vi "Vision Processing.vi"(4 "error in (no error)":errorcluster, 7 "Image Size":T3=enum."320x240") -> ()   [LabVIEW 2015]
uses:
  Vision Support Code/Camera Types.ctl
  <vilib>/Rock Robotics/WPI/Camera/WPI_CameraImageSize.ctl
  <vilib>/Rock Robotics/WPI/Camera/WPI_CameraExposure Values.ctl
  <vilib>/Rock Robotics/WPI/Camera/WPI_CameraFrameRate.ctl
  <vilib>/Rock Robotics/WPI/Camera/WPI_CameraWhite Balance Values.ctl
  <vilib>/Rock Robotics/Network Tables/NT Read Boolean.vi
  Robot Global Data.vi
  Global Variables/Vision Processing Data.vi
  <vilib>/vision/NI_Vision_Development_Module.lvlib
panel:
  out "Highest Avg Score":dbl
  in  "Min Score Threshold":i32=75
  out "Detected Targets":T1(array[cluster]) {"Normalized Rect"."Numeric 5" format="%#_2g"; "Normalized Rect"."Numeric 3" format="%#_2g"; "Normalized Rect"."Numeric 2" format="%#_2g"; "Normalized Rect"."Numeric" format="%#_2g"}
  out "Sorted Particle Scores":T2(array[cluster]) {"Moment Factor" format="%#_3g"; "Aspect Ratio" format="%#_3g"; "Area to CH" format="%#_3g"; "X" format="%#_3g"; "Y" format="%#_3g"}
  in  "Display Original":bool=TRUE
  in  "Display Mask":bool=TRUE
  out "fps":dbl
  in  "Emphasize Limit Tests":bool=TRUE
  in  "Camera Type":T4=enum."MS HD3000 square"
  in  "Aspect Fudge Factor":dbl=1.0
  in  "Score Threshold":dbl=75.0
  out "ms to process":u32
  out "Qualified Particles":i32
  in  "LED Color":T5={"Hue"={75.0, 175.0}, "Sat"={0.0, 255.0}, "Val"={50.0, 255.0}} {"Hue" scale=0.0..255.0 scale format="%#_3g"}
  out "Masked":T6(plugin-control)
  out "Original Image":T6(plugin-control)
  # "Density Profile"
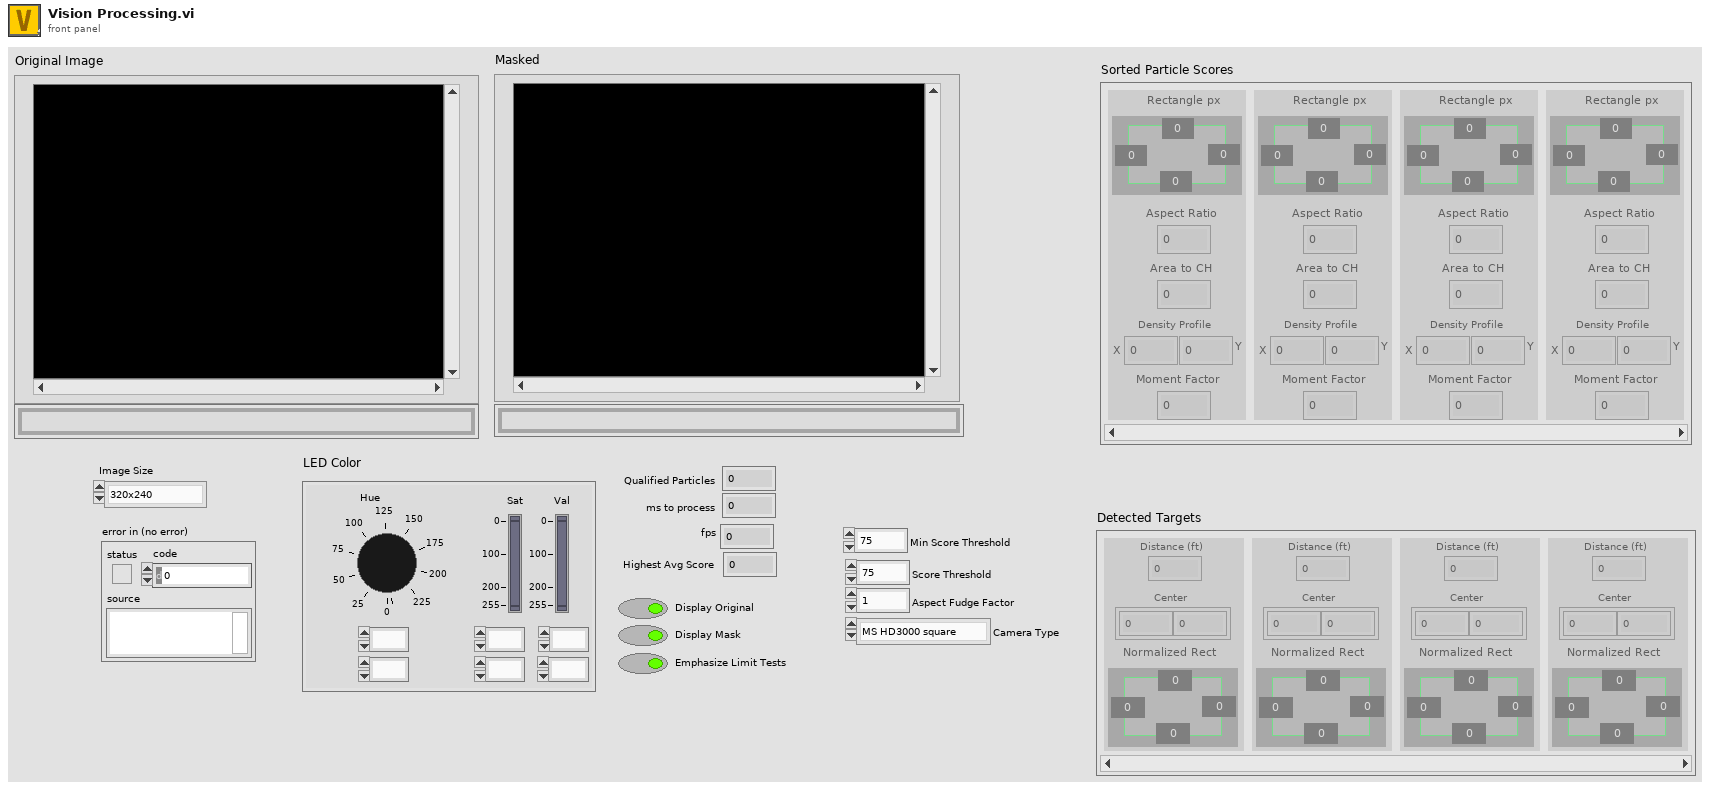
[diagram p1: front panel]
types:
  T1 = cluster{"Distance (ft)":dbl, "Center":cluster{dbl, dbl}, "Normalized Rect":cluster{"Numeric":dbl, "Numeric 2":dbl, "Numeric 3":dbl, "Numeric 5":dbl}}[]
  T2 = cluster{"Rectangle px":cluster{"Numeric":dbl, "Numeric 2":dbl, "Numeric 3":dbl, "Numeric 5":dbl}, "Aspect Ratio":dbl, "Area to CH":dbl, "X":dbl, "Y":dbl, "Moment Factor":dbl}[]
  T3 = typedef "WPI_CameraImageSize.ctl" = enum16{"640x480", "320x240", "160x120", "Custom"}
  T4 = typedef "Camera Types.ctl" = enum16{"206", "1011", "1013", "MS HD3000 square", "MS HD3000 640x480"}
  T5 = cluster{"Hue":cluster{dbl, dbl}, "Sat":cluster{dbl, dbl}, "Val":cluster{dbl, dbl}}
  T6 = typedef "IMAQ Image.ctl" = refnum<image>
  T7 = typedef "WPI_CameraWhite Balance Values.ctl" = enum16{"Auto", "Fixed indoor", "Fixed outdoor 1", "Fixed outdoor 2", "Fixed fluorescent 1", "Fixed fluorescent 2", "Hold current", "Custom"}
  T8 = typedef "WPI_CameraFrameRate.ctl" = u32
  T9 = typedef "WPI_CameraExposure Values.ctl" = enum16{"Auto", "Flicker-free 50 Hz", "Flicker-free 60 Hz", "Hold current", "Custom"}
  T10 = typedef "Particle Parameters" = i32
  T11 = typedef "Image Type" = u32
  T12 = typedef "WPI_CameraDevRef.ctl" = cluster{"Camera Address":string, "CameraStatus":errorcluster}
  T13 = cluster{"Bounding box":cluster{"left":dbl, "top":dbl, "right":dbl, "bottom":dbl}, "Aspect Ratio":dbl, "Area to CH":dbl, "X Mask":dbl, "Y Mask":dbl, "Moment":dbl}[]
  T14 = cluster{"Rectangle":cluster{"Numeric":dbl, "Numeric 2":dbl, "Numeric 3":dbl, "Numeric 5":dbl}, "L":dbl, "Area to CH":dbl, "X":dbl, "Y":dbl, "Moment Factor":dbl}[]
  T15 = cluster{"Distance (ft)":dbl, "Center":cluster{dbl, dbl}, "Normalized Rect":cluster{"Numeric":dbl, "Numeric 2":dbl, "Numeric 3":dbl, "Numeric 5":dbl}}
  T16 = cluster{"Rectangle":cluster{"Numeric":dbl, "Numeric 2":dbl, "Numeric 3":dbl, "Numeric 5":dbl}, "L":dbl, "Area to CH":dbl, "X":dbl, "Y":dbl, "Moment Factor":dbl}
  T17 = cluster{"Numeric":dbl, "Numeric 2":dbl, "Numeric 3":dbl, "Numeric 5":dbl}
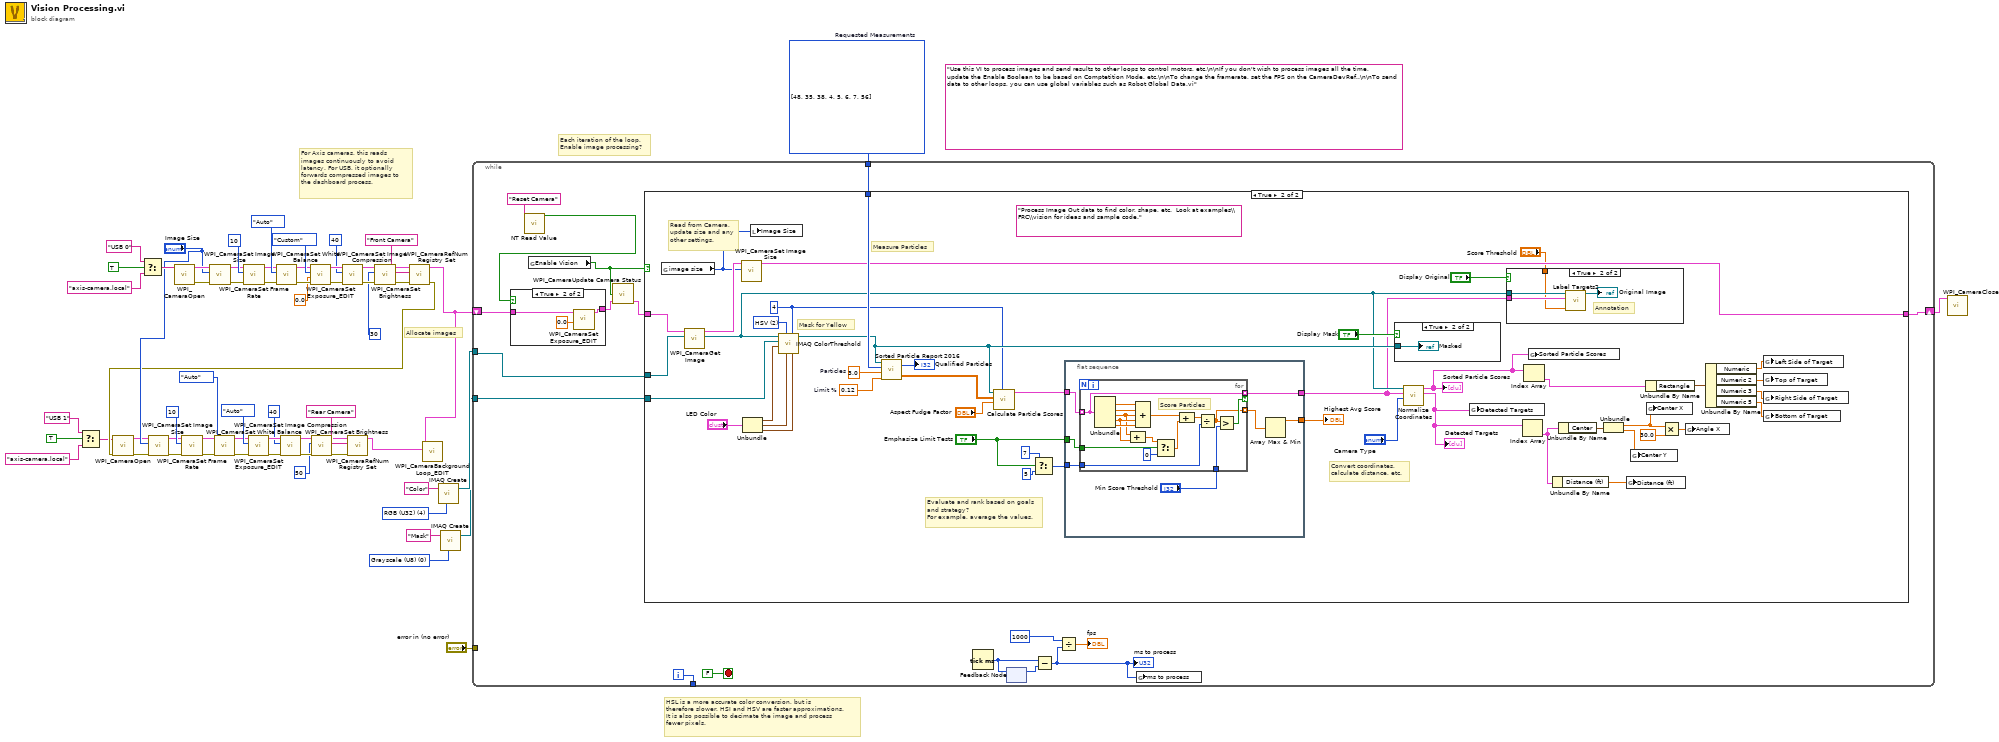
[diagram p0: block diagram]
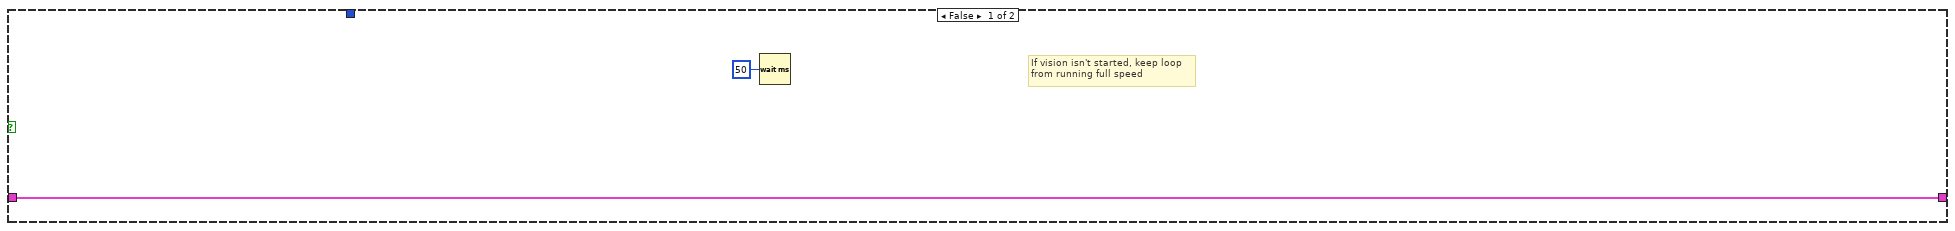
[diagram p3: hidden frame]
diagram:
  (unwired) "Use this VI to process images and send results to other loops to control motors, etc.\n\nIf you don't wish to process images all the time, update the Enable Boolean to be based on Comptetition Mode, etc.\n\nTo change the framerate, set the FPS on the CameraDevRef..\n\nTo send data to other loops, you can use global variables such as Robot Global Data.vi"
  w56 = T10[] [48, 35, 38, 4, 5, 6, 7, 56] items=["Center of Mass X", "Center of Mass Y", "First Pixel X", "First Pixel Y", "Bounding Rect Left", "Bounding Rect Top", "Bounding Rect Right", "Bounding Rect Bottom", "Max Feret Diameter Start X", "Max Feret Diameter Start Y", "Max Feret Diameter End X", "Max Feret Diameter End Y", "Max Horiz. Segment Length Left", "Max Horiz. Segment Length Right", "Max Horiz. Segment Length Row", "-", "Bounding Rect Width", "Bounding Rect Height", "Bounding Rect Diagonal", "Perimeter", "Convex Hull Perimeter", "Holes' Perimeter", "Max Feret Diameter", "Equivalent Ellipse Major Axis", "Equivalent Ellipse Minor Axis", "Equivalent Ellipse Minor Axis (Feret)", "Equivalent Rect Long Side", "Equivalent Rect Short Side", "Equivalent Rect Diagonal", "Equivalent Rect Short Side (Feret)", "Average Horiz. Segment Length", "Average Vert. Segment Length", "Hydraulic Radius", "Waddel Disk Diameter", "-", "Area", "Holes' Area", "Particle & Holes' Area", "Convex Hull Area", "Image Area", "-", "Number of Holes", "Number of Horiz. Segments", "Number of Vert. Segments", "-", "Orientation", "Max Feret Diameter Orientation", "-", "% Area/Image Area", "% Area/(Particle & Holes' Area)", "Ratio of Equivalent Ellipse Axes", "Ratio of Equivalent Rect Sides", "-", "Elongation Factor", "Compactness Factor", "Heywood Circularity Factor", "Type Factor", "-", "Sum X", "Sum Y", "Sum XX", "Sum XY", "Sum YY", "Sum XXX", "Sum XXY", "Sum XYY", "Sum YYY", "-", "Moment of Inertia XX", "Moment of Inertia XY", "Moment of Inertia YY", "Moment of Inertia XXX", "Moment of Inertia XXY", "Moment of Inertia XYY", "Moment of Inertia YYY", "Norm. Moment of Inertia XX", "Norm. Moment of Inertia XY", "Norm. Moment of Inertia YY", "Norm. Moment of Inertia XXX", "Norm. Moment of Inertia XXY", "Norm. Moment of Inertia XYY", "Norm. Moment of Inertia YYY", "Hu Moment 1", "Hu Moment 2", "Hu Moment 3", "Hu Moment 4", "Hu Moment 5", "Hu Moment 6", "Hu Moment 7"]  # Requested Measurements
  w59 = T11 0 items=["Grayscale (U8)", "Grayscale (I16)", "Grayscale (SGL)", "Complex (CSG)", "RGB (U32)", "HSL (U32)", "RGB (U64)", "Grayscale (U16)"] ("Image Type")
  w61 = T11 4 items=["Grayscale (U8)", "Grayscale (I16)", "Grayscale (SGL)", "Complex (CSG)", "RGB (U32)", "HSL (U32)", "RGB (U64)", "Grayscale (U16)"] ("Image Type")
  # "Each iteration of the loop,\nEnable image processing?"
  # "HSL is a more accurate color conversion, but is\ntherefore slower. HSI and HSV are faster approximations.\nIt is also possible to decimate the image and process\nfewer pixels."
  # "For Axis cameras, this reads\nimages continuously to avoid\nlatency. For USB, it optionally\nforwards compressed images to\nthe dashboard process."
  # "Allocate images"
  n1 = Select(t="USB 1" ("format string"), s=TRUE ("dot notation? (F)"), f="axis-camera.local" ("format string")) -> (s? t:f=w25:string)
  n2 = Select(t="USB 0" ("format string"), s=TRUE ("dot notation? (F)"), f="axis-camera.local" ("format string")) -> (s? t:f=w55:string)
  n3 = call <vilib>:"WPI_CameraOpen.vi"("Camera Address"=w55) -> ("error out"=w43:errorcluster, "CameraDevRef"=w42:T12)  [unwired: 1 in, 8 out]
  n4 = call <vilib>:"WPI_CameraSet Image Size.vi"("error in (no error)"=w43, "Image Size"="Image Size", "CameraDevRef"=w42) -> ("error out"=w44:errorcluster, "CameraDevRef Out"=w41:T12)  [unwired: 1 in, 6 out]
  n5 = call <vilib>:"WPI_CameraSet Frame Rate.vi"("error in (no error)"=w44, "Frame Rate (fps)"=T8 10, "CameraDevRef"=w41) -> ("error out"=w45:errorcluster, "CameraDevRef Out"=w39:T12)  [unwired: 7 out]
  n6 = call <vilib>:"WPI_CameraSet White Balance.vi"("error in (no error)"=w45, "White Balance"=WPI_CameraWhite_Balance_Values."Auto", "CameraDevRef"=w39) -> ("error out"=w46:errorcluster, "CameraDevRef Out"=w40:T12)  [unwired: 1 in, 6 out]
  n7 = call "WPI_CameraSet Exposure_EDIT.vi"("error in (no error)"=w46, "Exposure (%)"=0.0, "Exposure"=WPI_CameraExposure_Values."Custom", "CameraDevRef"=w40) -> ("error out"=w47:errorcluster, "CameraDevRef Out"=w37:T12)  [unwired: 6 out]
  n8 = call <vilib>:"WPI_CameraSet Image Compression.vi"("error in (no error)"=w47, "Compression"=40, "CameraDevRef"=w37) -> ("error out"=w48:errorcluster, "CameraDevRef Out"=w38:T12)  [unwired: 7 out]
  n9 = call <vilib>:"WPI_CameraSet Brightness.vi"("error in (no error)"=w48, "Brightness"=30, "CameraDevRef"=w38) -> ("error out"=w49:errorcluster, "CameraDevRef Out"=w31:T12)  [unwired: 7 out]
  n10 = call <vilib>:"WPI_CameraRefNum Registry Set.vi"("error in (no error)"=w49, "refnum name"="Front Camera", "CameraDevRef"=w31) -> ("error out"=w28:errorcluster, "CameraDevRef"=w26:T12)  [unwired: 1 in, 6 out]
  n11 = call <vilib>:"WPI_CameraOpen.vi"("error in (no error)"=w28, "Camera Address"=w25) -> ("error out"=w14:errorcluster, "CameraDevRef"=w13:T12)  [unwired: 8 out]
  n12 = call <vilib>:"WPI_CameraSet Image Size.vi"("error in (no error)"=w14, "Image Size"="Image Size", "CameraDevRef"=w13) -> ("error out"=w15:errorcluster, "CameraDevRef Out"=w12:T12)  [unwired: 1 in, 6 out]
  n13 = call <vilib>:"WPI_CameraSet Frame Rate.vi"("error in (no error)"=w15, "Frame Rate (fps)"=T8 10, "CameraDevRef"=w12) -> ("error out"=w16:errorcluster, "CameraDevRef Out"=w10:T12)  [unwired: 7 out]
  n14 = call <vilib>:"WPI_CameraSet White Balance.vi"("error in (no error)"=w16, "White Balance"=WPI_CameraWhite_Balance_Values."Auto", "CameraDevRef"=w10) -> ("error out"=w17:errorcluster, "CameraDevRef Out"=w11:T12)  [unwired: 1 in, 6 out]
  n15 = call "WPI_CameraSet Exposure_EDIT.vi"("error in (no error)"=w17, "Exposure"=WPI_CameraExposure_Values."Auto", "CameraDevRef"=w11) -> ("error out"=w18:errorcluster, "CameraDevRef Out"=w8:T12)  [unwired: 1 in, 6 out]
  n16 = call <vilib>:"WPI_CameraSet Image Compression.vi"("error in (no error)"=w18, "Compression"=40, "CameraDevRef"=w8) -> ("error out"=w19:errorcluster, "CameraDevRef Out"=w9:T12)  [unwired: 7 out]
  n17 = call <vilib>:"WPI_CameraSet Brightness.vi"("error in (no error)"=w19, "Brightness"=50, "CameraDevRef"=w9) -> ("error out"=w20:errorcluster, "CameraDevRef Out"=w4:T12)  [unwired: 7 out]
  n18 = call <vilib>:"WPI_CameraRefNum Registry Set.vi"("error in (no error)"=w20, "refnum name"="Rear Camera", "CameraDevRef"=w4) -> ("CameraDevRef"=w1:T12)  [unwired: 1 in, 7 out]
  n19 = call "WPI_CameraBackground Loop_EDIT.vi"("Front CameraDevRef"=w26, "Rear CameraDevRef"=w1) -> ()  [unwired: 9 in]
  n20 = call "IMAQ Create"("Image Name"="Color", "Image Type"=w61) -> ("New Image"=w60:T6)  [unwired: 2 in, 2 out]
  n21 = call "IMAQ Create"("Image Name"="Mask", "Image Type"=w59) -> ("New Image"=w57:T6)  [unwired: 2 in, 2 out]
  n22 = while {
    tunnel: w60 -> [w66]
    tunnel: w57 -> [w78]
    tunnel: w56 -> [w77]
    tunnel: "error in (no error)" -> [_]
    tunnel: [w74] -> _
    shift-right: [w72] -> w32
    shift-left: w26 -> [w68]
    i -> [w74]
    stop <- FALSE stop-if-true
    n23 = call-poly <vilib>:"NT Read Value.vi"("Name"="Reset Camera") -> ("Boolean"=w65:bool)  [unwired: 9 in, 1 out]
    n24 = case shown="True" w65 {
      tunnel: w68 -> [w80 w83]
      tunnel: [w80 w82] -> w67
      frame False {
      }
      frame True {
        n25 = call "WPI_CameraSet Exposure_EDIT.vi"("Exposure (%)"=0.0, "CameraDevRef"=w83) -> ("CameraDevRef Out"=w82:T12)  [unwired: 2 in, 7 out]
      }
    }
    n26 = global read "Robot Global Data.vi" "Enable Vision"() -> (w63:bool)
    n27 = call <vilib>:"WPI_CameraUpdate Camera Status.vi"("CameraDevRef In"=w67, "Enable Vision"=w63) -> ("CameraDevRef Out"=w73:T12)  [unwired: 3 in]
    n28 = case shown="True" w63 {
      tunnel: w78 -> [_ w131]
      tunnel: w77 -> [_ w126]
      tunnel: w73 -> [w84 w122]
      tunnel: w66 -> [_ w121]
      tunnel: [w84 w119] -> w72
      frame False {
        # "If vision isn't started, keep loop\nfrom running full speed"
        n29 = Wait (ms)(milliseconds to wait=u32 50) -> ()  [unwired: 1 out]
      }
      frame True {
        w103 = 4 ("Replace Value")
        w116 = u16 2 items=["RGB", "HSL", "HSV", "HSI"] ("Color Mode")
        (unwired) "Process Image Out data to find color, shape, etc.  Look at examples\\FRC\\vision for ideas and sample code."
        w123 = 0.12  # Limit %
        w125 = 3.0  # Particles
        # "Evaluate and rank based on goals\nand strategy?\nFor example, average the values."
        # "Read from Camera,\nupdate size and any\nother settings."
        # "Measure Particles"
        # "Convert coordinates,\ncalculate distance, etc."
        # "Mask for Yellow"
        n30 = global read "Robot Global Data.vi" "image size"() -> (w102:T3)
        n31 = call <vilib>:"WPI_CameraGet Image.vi"("Image"=w121, "CameraDevRef"=w122) -> ("Image Out"=w106:T6, "CameraDevRef Out"=w120:T12)  [unwired: 7 in, 1 out]
        n32 = call <vilib>:"WPI_CameraSet Image Size.vi"("Image Size"=w102, "CameraDevRef"=w120) -> ("CameraDevRef Out"=w119:T12)  [unwired: 2 in, 7 out]
        n33 = Unbundle("LED Color") -> ("Hue"=w130:cluster{dbl, dbl}, "Sat"=w129:cluster{dbl, dbl}, "Val"=w128:cluster{dbl, dbl})
        n34 = local write "Image Size"(w102) -> ()
        n35 = call "IMAQ ColorThreshold"("Blue or Luma or Val or Inten Range"=w128, "Replace Value"=w103, "Green or Sat Range"=w129, "Color Mode"=w116, "Red or Hue Range"=w130, "Image Dst"=w131, "Image Src"=w106) -> ("Image Dst Out"=w115:T6)  [unwired: 3 in, 1 out]
        n36 = call "Sorted Particle Report 2016.vi"("Min Area Size %"=w123, "Particle Count Limit"=w125, "Pixel Measurements"=w126, "Image in"=w115) -> ("Sorted Data"=w114:dbl[][], "Particles"=→"Qualified Particles":i32)
        n37 = call "Calculate Particle Scores.vi"("Pixel Value"=w103, "Aspect Fudge Factor"="Aspect Fudge Factor", "Sorted Data"=w114, "Image in"=w115) -> ("Scores"=w112:T13)  [unwired: 7 in]
        n38 = Select(t=7, s="Emphasize Limit Tests", f=5) -> (s? t:f=w109:i32)
        n39 = flat-sequence {
          tunnel: w112 -> [w142]
          tunnel: w109 -> [w140]
          tunnel: [w143] -> w108
          tunnel: [w137] -> w105
          tunnel: "Emphasize Limit Tests" -> [w141]
          frame #0 {
            n40 = for {
              tunnel: w142 -> [w157] mode=indexing
              tunnel: [w157] -> w137 mode=indexing if=w156
              tunnel: [w155] -> w138 mode=indexing
              tunnel: w140 -> [w154]
              tunnel: "Min Score Threshold" -> [w153]
              tunnel: w141 -> [w146]
              # "Score Particles"
              n41 = Unbundle(w157) -> ("Aspect Ratio"=w159:dbl, "Area to CH"=w158:dbl, "X Mask"=w148:dbl, "Y Mask"=w149:dbl, "Moment"=w150:dbl)  [unwired: 1 out]
              n42 = Compound Arithmetic op=ADD(w148, w149) -> (w147:dbl)
              n43 = Compound Arithmetic op=ADD(w159, w158, w148, w149, w150) -> (w152:dbl)
              n44 = Select(t=w147, s=w146, f=0) -> (s? t:f=w145:dbl)
              n45 = Compound Arithmetic op=ADD(w152, w145) -> (w151:dbl)
              n46 = Divide(x=w151, y=w154) -> (x/y=w155:dbl)
              n47 = Greater?(x=w155, y=w153) -> (0:w156:bool)
            }
            n48 = Array Max & Min(array=w138) -> (max value=w143:dbl)  [unwired: 3 out]
          }
        }
        n49 = case shown="True" "Display Mask" {
          tunnel: w115 -> [_ w136]
          frame False {
          }
          frame True {
            "Masked" <- w136
          }
        }
        n50 = call "Normalize Coordinates.vi"("Camera Type"="Camera Type", "Targets"=w105, "Image in"=w106) -> ("Found Targets"=w97:T1, "Sorted Scores"=w95:T14)  [unwired: 6 in, 1 out]
        "Sorted Particle Scores" <- w95
        "Detected Targets" <- w97
        n51 = global write "Vision Processing Data.vi" "Detected Targets"(w97) -> ()
        n52 = case shown="True" "Display Original" {
          tunnel: w106 -> [_ w135]
          tunnel: w105 -> [_ w134]
          tunnel: "Score Threshold" -> [_ w133]
          frame False {
          }
          frame True {
            # "Annotation"
            n53 = call "Label Targets2.vi"("Score Threshold"=w133, "Targets"=w134, "Image in"=w135) -> ("Image out"=→"Original Image":T6)  [unwired: 8 in]
          }
        }
        n54 = Index Array(array=w97) -> (element=w87:T15)  [unwired: 1 in]
        n55 = Index Array(array=w95) -> (element=w100:T16)  [unwired: 1 in]
        n56 = global write "Vision Processing Data.vi" "Sorted Particle Scores"(w95) -> ()
        n57 = Unbundle By Name(w87) -> ("Distance (ft)"=w86:dbl)
        n58 = Unbundle By Name(w87) -> ("Center"=w98:cluster{dbl, dbl})
        n59 = Unbundle(w98) -> (w94:dbl, w92:dbl)
        n60 = global write "Vision Processing Data.vi" "Distance (ft)"(w86) -> ()
        n61 = global write "Vision Processing Data.vi" "Center Y"(w92) -> ()
        n62 = Unbundle By Name(w100) -> ("Rectangle"=w99:T17)
        n63 = global write "Vision Processing Data.vi" "Center X"(w94) -> ()
        n64 = Multiply(x=w94, y=30.0) -> (x*y=w93:dbl)
        n65 = global write "Vision Processing Data.vi" "Angle X"(w93) -> ()
        n66 = Unbundle By Name(w99) -> ("Numeric"=w88:dbl, "Numeric 2"=w89:dbl, "Numeric 3"=w90:dbl, "Numeric 5"=w91:dbl)
        n67 = global write "Vision Processing Data.vi" "Left Side of Target"(w88) -> ()
        n68 = global write "Vision Processing Data.vi" "Top of Target"(w89) -> ()
        n69 = global write "Vision Processing Data.vi" "Right Side of Target"(w90) -> ()
        n70 = global write "Vision Processing Data.vi" "Bottom of Target"(w91) -> ()
        "Highest Avg Score" <- w108
      }
    }
    n71 = Tick Count (ms)() -> (millisecond timer value=w75:u32)
    n72 = feedback-in #1(w75) -> ()
    n73 = feedback #1() -> (w76:u32)  [unwired: 1 in]
    n74 = Subtract(x=w75, y=w76) -> (x-y=w71:u32)
    "ms to process" <- w71
    n75 = Divide(x=1000 ("Brightness"), y=w71) -> (x/y=→"fps":dbl)
    n76 = global write "Robot Global Data.vi" "ms to process"(w71) -> ()
  }
  n77 = call <vilib>:"WPI_CameraClose.vi"("CameraDevRef"=w32) -> ()  [unwired: 1 in, 10 out]
